vi "Battery_Charger 1.vi"() -> ()   [LabVIEW 2015]
uses:
  Battery_Charger_variables.vi
  <vilib>/Utility/NIReport.llb/NI_report.lvclass
  <instrlib>/Agilent N6700 Series/Agilent N6700 Series.lvlib
  <vilib>/addons/_office/NI_ReportGenerationToolkit.lvlib
panel:
  out "Charged":bool
  in  "Stop":bool
  out "Voltage Graph":dbl[](graph)
  out "Voltage Measurement":dbl format="%^.3e"
  out "Current Measurement":dbl format="%^.3e"
  out "Count":i32
  out "Current Graph":dbl[](graph)
  in  "report file path":path
  in  "Start":bool
  in  "VISA resource name":refnum<visa-resource-name>="USB0::0x0957::0x0F07::MY53002228::INSTR"
  in  "Channel Name (1)":string="4"
  in  "Positive Voltage Limit  (5.0 V)":dbl=5.0 format="%^.3e"
  in  "Negative Voltage Limit (0.0 volts)":dbl format="%^.3e"
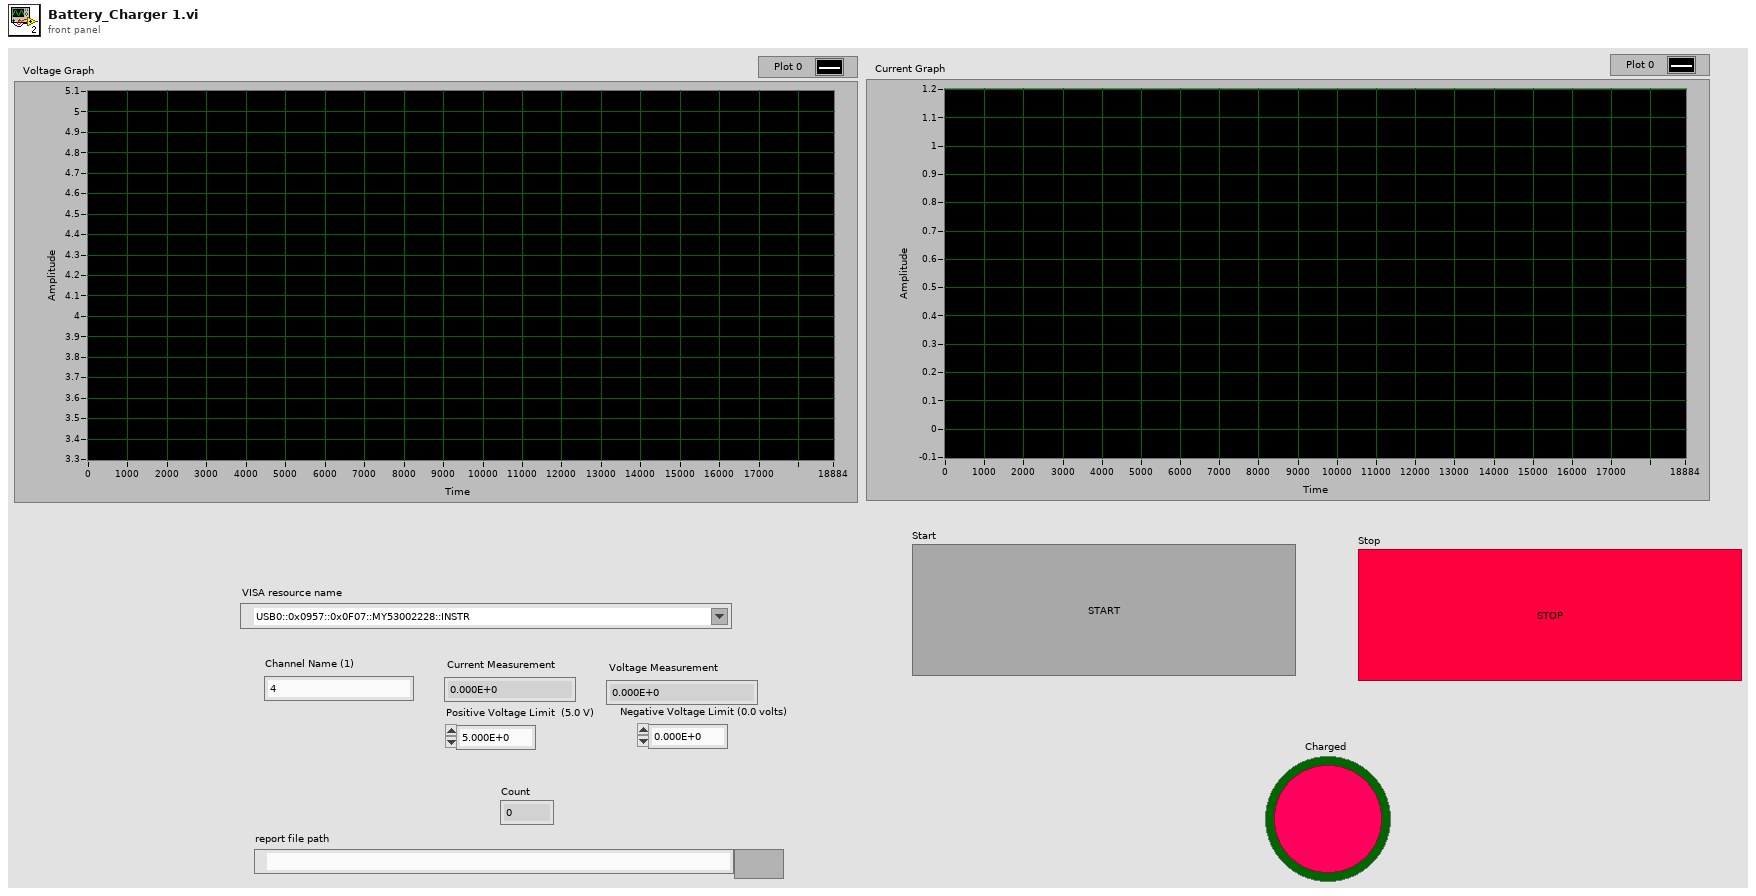
[diagram p1: front panel]
types:
  T1 = enum16{"Standard Report", "HTML", "Word", "Excel"}
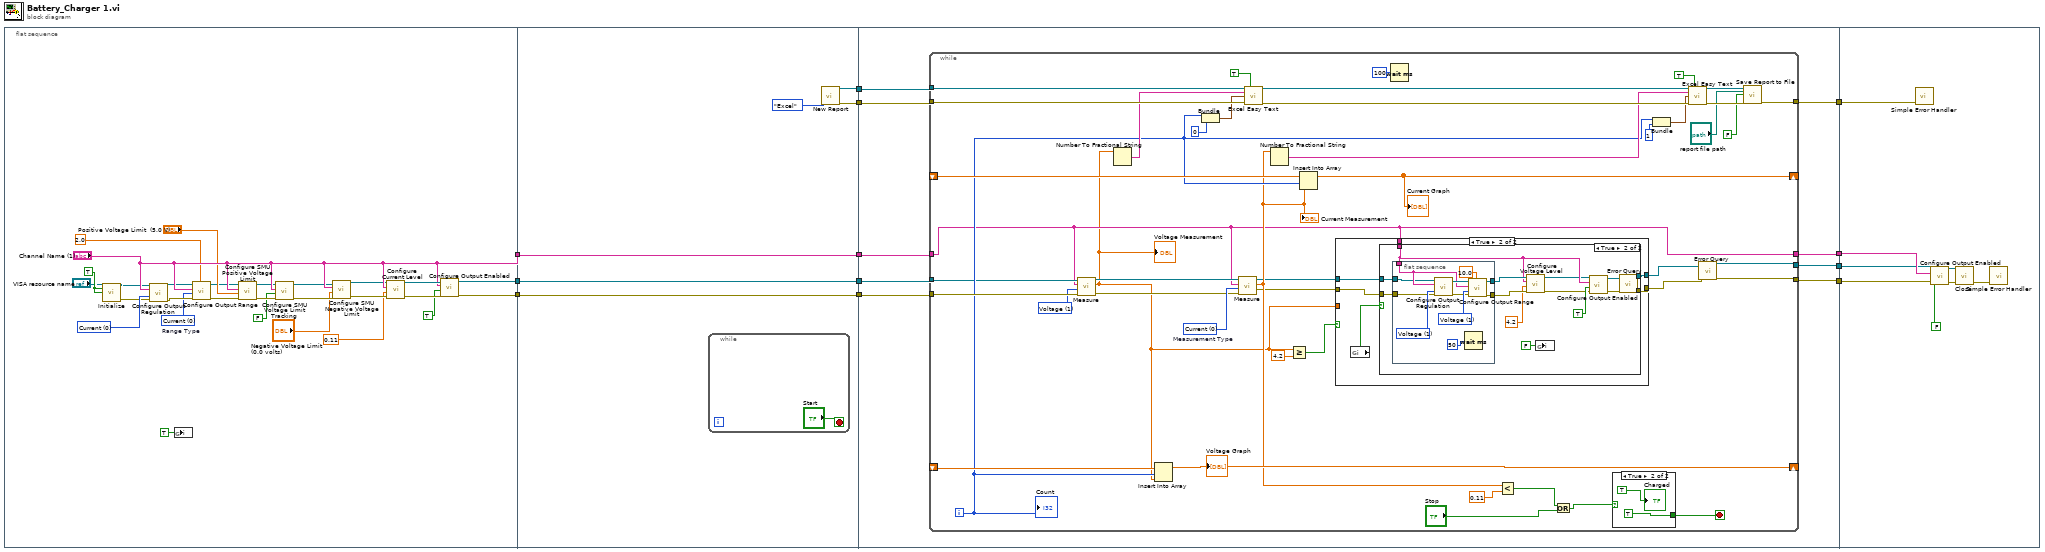
[diagram p0: block diagram]
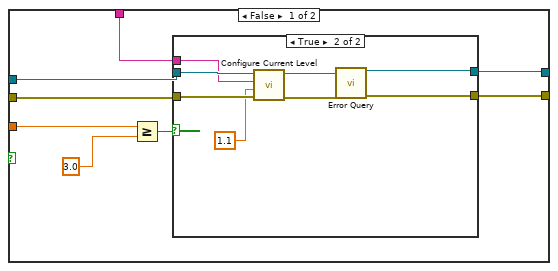
[diagram p2: hidden frame]
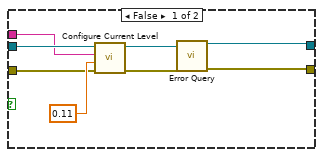
[diagram p3: hidden frame]
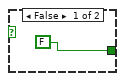
[diagram p5: hidden frame]
diagram:
  n1 = flat-sequence {
    tunnel: ["Channel Name (1)"] -> w12
    tunnel: [w38] -> w11
    tunnel: [w37] -> w10
    tunnel: [w46] -> w9
    tunnel: w12 -> [w46]
    tunnel: [w45] -> w8
    tunnel: w11 -> [w45]
    tunnel: [w44] -> w7
    tunnel: w10 -> [w44]
    tunnel: [w42] -> w6
    tunnel: [w41] -> w5
    tunnel: w9 -> [w56]
    tunnel: w8 -> [w55]
    tunnel: w7 -> [w54]
    tunnel: [w53] -> w2
    tunnel: [w52] -> w3
    tunnel: [w51] -> w4
    tunnel: w6 -> [w50]
    tunnel: w5 -> [w49]
    tunnel: [w48] -> w1
    tunnel: w4 -> [w165]
    tunnel: w3 -> [w163]
    tunnel: w2 -> [w162]
    tunnel: w1 -> [w164]
    frame #0 {
      w24 = 0 items=["Voltage"=1, "Current"=0] ("Priority (1: Voltage)")
      w27 = TRUE ("Reset? (T: Yes)")
      w26 = 0 items=["Voltage"=1, "Current"=0]  # Range Type
      n2 = call <instrlib>:"Initialize.vi"("VISA resource name"="VISA resource name", "ID Query? (T: Yes)"=w27, "Reset? (T: Yes)"=w27) -> ("VISA resource name out"=w16:refnum<visa-resource-name>, "error out"=w15:errorcluster)  [unwired: 11 in]
      n3 = call <instrlib>:"Configure Output Regulation.vi"("VISA resource name"=w16, "Channel Name (1)"="Channel Name (1)", "Output Regulation Priority (1: Voltage)"=w24, "error in (no error)"=w15) -> ("VISA resource name out"=w28:refnum<visa-resource-name>, "error out"=w29:errorcluster)  [unwired: 10 in]
      n4 = global write "Battery_Charger_variables.vi" "i"(TRUE ("i")) -> ()
      n5 = call <instrlib>:"Configure Output Range.vi"("Range (0.0)"=2.0, "error in (no error)"=w29, "Range Type (1: Voltage)"=w26, "Channel Name (1)"="Channel Name (1)", "VISA resource name"=w28) -> ("error out"=w31:errorcluster, "VISA resource name out"=w30:refnum<visa-resource-name>)  [unwired: 5 in]
      n6 = call <instrlib>:"Configure SMU Positive Voltage Limit.vi"("error in (no error)"=w31, "Positive Voltage Limit (0.0 volts)"="Positive Voltage Limit  (5.0 V)", "Channel Name (1)"="Channel Name (1)", "VISA resource name"=w30) -> ("error out"=w33:errorcluster, "VISA resource name out"=w32:refnum<visa-resource-name>)  [unwired: 6 in]
      n7 = call <instrlib>:"Configure SMU Voltage Limit Tracking.vi"("error in (no error)"=w33, "Enable Voltage Limit Tracking (False)"=FALSE, "Channel Name (1)"="Channel Name (1)", "VISA resource name"=w32) -> ("error out"=w20:errorcluster, "VISA resource name out"=w21:refnum<visa-resource-name>)  [unwired: 6 in]
      n8 = call <instrlib>:"Configure SMU Negative Voltage Limit.vi"("error in (no error)"=w20, "Negative Voltage Limit (0.0 volts)"="Negative Voltage Limit (0.0 volts)", "Channel Name (1)"="Channel Name (1)", "VISA resource name"=w21) -> ("error out"=w17:errorcluster, "VISA resource name out"=w18:refnum<visa-resource-name>)  [unwired: 6 in]
      n9 = call <instrlib>:"Configure Current Level.vi"("error in (no error)"=w17, "Level  (0.0 A)"=0.11, "Channel Name (1)"="Channel Name (1)", "VISA resource name"=w18) -> ("error out"=w39:errorcluster, "VISA resource name out"=w40:refnum<visa-resource-name>)  [unwired: 6 in]
      n10 = call <instrlib>:"Configure Output Enabled.vi"("error in (no error)"=w39, "Enable Output (False)"=TRUE, "Channel Name (1)"="Channel Name (1)", "VISA resource name"=w40) -> ("error out"=w37:errorcluster, "VISA resource name out"=w38:refnum<visa-resource-name>)  [unwired: 6 in]
    }
    frame #1 {
      n11 = while {
        stop <- "Start" stop-if-true
      }
      n12 = call <vilib>:"New Report.vi"("report type"=T1."Excel") -> ("report out"=w42:refnum<class "NI_report.lvclass">, "error out"=w41:errorcluster)  [unwired: 13 in]
    }
    frame #2 {
      n13 = while {
        tunnel: w56 -> [w58]
        tunnel: w55 -> [w68]
        tunnel: w54 -> [w77]
        tunnel: [w86] -> w53
        tunnel: [w87] -> w52
        tunnel: [w58] -> w51
        tunnel: w50 -> [w99]
        tunnel: w49 -> [w98]
        tunnel: [w83] -> w48
        shift-right: [w89] -> _
        shift-left: _ -> [w88]
        shift-right: [w72] -> _
        shift-left: _ -> [w74]
        i -> [w73]
        stop <- w100 stop-if-true
        w76 = 1 items=["Current", "Voltage", "Power"] ("Measurement Type (1: Voltage)")
        w101 = 0 items=["Voltage"=1, "Current"=0]  # Measurement Type
        n14 = call <instrlib>:"Measure.vi"("error in (no error)"=w77, "Measurement Type (1: Voltage)"=w76, "Channel Name (1)"=w58, "VISA resource name"=w68) -> ("error out"=w79:errorcluster, "Measurement"=w57:dbl, "VISA resource name out"=w78:refnum<visa-resource-name>)  [unwired: 5 in]
        "Voltage Measurement" <- w57
        n15 = Number To Fractional String(number=w57) -> (F-format string=w75:string)  [unwired: 3 in]
        n16 = Insert Into Array(array=w74, index=w73, new element=w57) -> (w72:dbl[])
        "Voltage Graph" <- w72
        n17 = Bundle(w73, "offset (0)"=0) -> (w97:cluster{i32, "offset (0)":i32})  [unwired: 1 in]
        n18 = call <instrlib>:"Measure.vi"("error in (no error)"=w79, "Measurement Type (1: Voltage)"=w101, "Channel Name (1)"=w58, "VISA resource name"=w78) -> ("error out"=w61:errorcluster, "Measurement"=w66:dbl, "VISA resource name out"=w62:refnum<visa-resource-name>)  [unwired: 5 in]
        "Current Measurement" <- w66
        n19 = call <vilib>:"Excel Easy Text.vi"("report in"=w99, "border? (F)"=TRUE, "text"=w75, "start (-1, -1)"=w97, "error in (no error)"=w98) -> ("report out"=w94:refnum<class "NI_report.lvclass">, "error out"=w95:errorcluster)  [unwired: 6 in, 3 out]
        n20 = Number To Fractional String(number=w66) -> (F-format string=w91:string)  [unwired: 3 in]
        n21 = Greater Or Equal?(x=w57, y=4.2) -> (x >= y?=w64:bool)
        n22 = Insert Into Array(array=w88, index=w73, new element=w66) -> (w89:dbl[])
        "Current Graph" <- w89
        n23 = case shown="True" w64 {
          tunnel: w62 -> [w106 w128]
          tunnel: w61 -> [w105 w127]
          tunnel: w58 -> [w104 w129]
          tunnel: [w103 w130] -> w60
          tunnel: [w102 w131] -> w59
          tunnel: w57 -> [w108 _]
          frame False {
            n24 = Greater Or Equal?(x=w108, y=3.0) -> (x >= y?=w109:bool)
            n25 = case shown="True" w109 {
              tunnel: w106 -> [w113 w125]
              tunnel: w105 -> [w114 w124]
              tunnel: w104 -> [w112 w123]
              tunnel: [w111 w120] -> w103
              tunnel: [w110 w119] -> w102
              frame False {
                n26 = call <instrlib>:"Configure Current Level.vi"("error in (no error)"=w114, "Level  (0.0 A)"=0.11, "Channel Name (1)"=w112, "VISA resource name"=w113) -> ("error out"=w116:errorcluster, "VISA resource name out"=w117:refnum<visa-resource-name>)  [unwired: 6 in]
                n27 = call <instrlib>:"Error Query.vi"("VISA resource name"=w117, "error in (no error)"=w116) -> ("VISA resource name out"=w111:refnum<visa-resource-name>, "error out"=w110:errorcluster)  [unwired: 10 in, 2 out]
              }
              frame True {
                n28 = call <instrlib>:"Configure Current Level.vi"("error in (no error)"=w124, "Level  (0.0 A)"=1.1, "Channel Name (1)"=w123, "VISA resource name"=w125) -> ("error out"=w121:errorcluster, "VISA resource name out"=w122:refnum<visa-resource-name>)  [unwired: 6 in]
                n29 = call <instrlib>:"Error Query.vi"("VISA resource name"=w122, "error in (no error)"=w121) -> ("VISA resource name out"=w120:refnum<visa-resource-name>, "error out"=w119:errorcluster)  [unwired: 10 in, 2 out]
              }
            }
          }
          frame True {
            n30 = global read "Battery_Charger_variables.vi" "i"() -> (w126:bool)
            n31 = case shown="True" w126 {
              tunnel: [w132 w145] -> w131
              tunnel: [w133 w144] -> w130
              tunnel: w129 -> [_ w139]
              tunnel: w128 -> [w133 w136]
              tunnel: w127 -> [w132 w135]
              frame False {
              }
              frame True {
                n32 = flat-sequence {
                  tunnel: w139 -> [w155]
                  tunnel: [w154] -> w141
                  tunnel: [w153] -> w142
                  tunnel: w136 -> [w151]
                  tunnel: w135 -> [w150]
                  frame #0 {
                    w156 = 1 items=["Voltage"=1, "Current"=0] ("Range Type (1: Voltage)")
                    w157 = 1 items=["Voltage"=1, "Current"=0] ("Output Regulation Priority (1: Voltage)")
                    n33 = call <instrlib>:"Configure Output Regulation.vi"("VISA resource name"=w151, "Channel Name (1)"=w155, "Output Regulation Priority (1: Voltage)"=w157, "error in (no error)"=w150) -> ("VISA resource name out"=w158:refnum<visa-resource-name>, "error out"=w149:errorcluster)  [unwired: 10 in]
                    n34 = Wait (ms)(milliseconds to wait=u32 50) -> ()  [unwired: 1 out]
                    n35 = call <instrlib>:"Configure Output Range.vi"("Range (0.0)"=10.0, "error in (no error)"=w149, "Range Type (1: Voltage)"=w156, "Channel Name (1)"=w155, "VISA resource name"=w158) -> ("error out"=w153:errorcluster, "VISA resource name out"=w154:refnum<visa-resource-name>)  [unwired: 5 in]
                  }
                }
                n36 = call <instrlib>:"Configure Voltage Level.vi"("error in (no error)"=w142, "Level  (0.0 volts)"=4.2, "Channel Name (1)"=w139, "VISA resource name"=w141) -> ("error out"=w137:errorcluster, "VISA resource name out"=w138:refnum<visa-resource-name>)  [unwired: 6 in]
                n37 = global write "Battery_Charger_variables.vi" "i"(FALSE ("i")) -> ()
                n38 = call <instrlib>:"Configure Output Enabled.vi"("error in (no error)"=w137, "Enable Output (False)"=TRUE, "Channel Name (1)"=w139, "VISA resource name"=w138) -> ("error out"=w146:errorcluster, "VISA resource name out"=w147:refnum<visa-resource-name>)  [unwired: 6 in]
                n39 = call <instrlib>:"Error Query.vi"("VISA resource name"=w147, "error in (no error)"=w146) -> ("VISA resource name out"=w144:refnum<visa-resource-name>, "error out"=w145:errorcluster)  [unwired: 10 in, 2 out]
              }
            }
          }
        }
        n40 = Wait (ms)(milliseconds to wait=u32 100) -> ()  [unwired: 1 out]
        n41 = Less?(x=w66, y=0.11) -> (x < y?=w67:bool)
        n42 = Or(x=w67, y="Stop") -> (x .or. y?=w70:bool)
        n43 = case shown="True" w70 {
          tunnel: [FALSE TRUE ("stop")] -> w100
          frame False {
          }
          frame True {
            "Charged" <- TRUE
          }
        }
        n44 = Bundle(w73, "offset (0)"=1) -> (w92:cluster{i32, "offset (0)":i32})  [unwired: 1 in]
        n45 = call <vilib>:"Excel Easy Text.vi"("report in"=w94, "border? (F)"=TRUE, "text"=w91, "start (-1, -1)"=w92, "error in (no error)"=w95) -> ("report out"=w85:refnum<class "NI_report.lvclass">, "error out"=w84:errorcluster)  [unwired: 6 in, 3 out]
        n46 = call <instrlib>:"Error Query.vi"("VISA resource name"=w60, "error in (no error)"=w59) -> ("VISA resource name out"=w87:refnum<visa-resource-name>, "error out"=w86:errorcluster)  [unwired: 10 in, 2 out]
        n47 = call-dynamic "Save Report to File.vi"("report in"=w85, "report file path"="report file path", "prompt to replace? (F)"=FALSE, "error in (no error)"=w84) -> ("error out"=w83:errorcluster)  [unwired: 10 in, 1 out]
        "Count" <- w73
      }
    }
    frame #3 {
      n48 = call <vilib>:"Simple Error Handler.vi"("error in (no error)"=w164) -> ()  [unwired: 1 in, 8 out]
      n49 = call <instrlib>:"Configure Output Enabled.vi"("error in (no error)"=w162, "Enable Output (False)"=FALSE, "Channel Name (1)"=w165, "VISA resource name"=w163) -> ("error out"=w167:errorcluster, "VISA resource name out"=w168:refnum<visa-resource-name>)  [unwired: 6 in]
      n50 = call <instrlib>:"Close.vi"("VISA resource name"=w168, "error in (no error)"=w167) -> ("error out"=w169:errorcluster)  [unwired: 13 in]
      n51 = call <vilib>:"Simple Error Handler.vi"("error in (no error)"=w169) -> ()  [unwired: 4 in, 5 out]
    }
  }
